vi "Read Channel Names.vi"(8 "error in (no error)":errorcluster, 11 "Temp Control in":refnum<class "Temp Control.lvclass">) -> (0 "error out":errorcluster, 2 "Channel Names":string[](array[string])=["Telescope RA", "Telescope DEC", "Telescope Moving?", "Telescope Status"], 3 "Temp Control out":refnum<class "Temp Control.lvclass">)   [LabVIEW 2022 SP3, in "Temp Control.lvclass"]
uses:
  Temp Control.lvclass
  Temp Control.lvclass/Temp Control.ctl
  hk-channel-class/hk-channel-class/HK Item/HK Item.lvclass
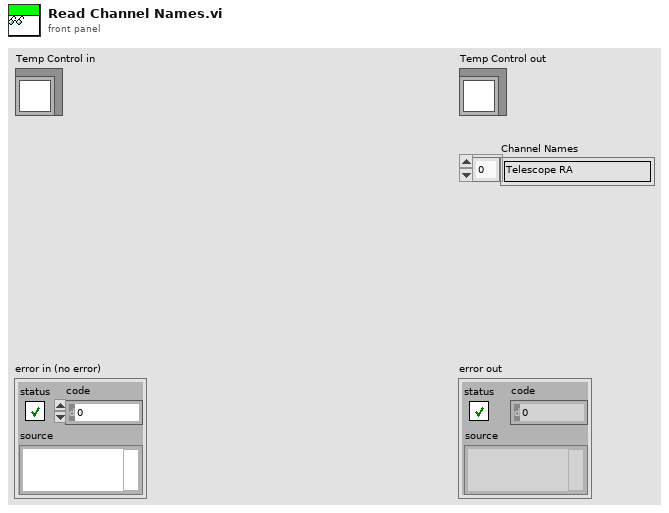
[diagram p1: front panel]
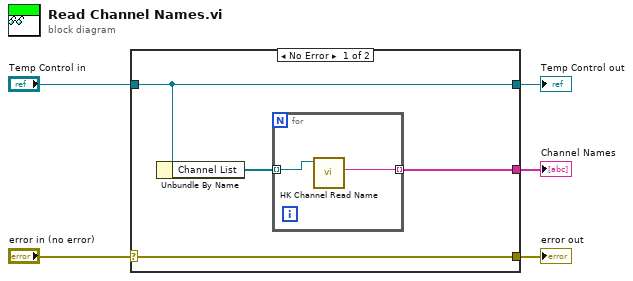
[diagram p0: block diagram]
diagram:
  n1 = case shown="No Error" "error in (no error)" {
    selector: "error in (no error)" -> [w9 w12]
    tunnel: [w9 w12] -> w4
    tunnel: [w8 w13] -> w2
    tunnel: "Temp Control in" -> [w8 w13]
    tunnel: [w6 _] -> w1
    frame No Error {
      n2 = Unbundle By Name(w8) -> ("Channel List"=w7:refnum<class "HK Item.lvclass">[])
      n3 = for {
        tunnel: w7 -> [w11] mode=indexing
        tunnel: [w10] -> w6 mode=indexing
        n4 = call "HK Channel Read Name.vi"("HK Item in"=w11) -> ("Name"=w10:string)  [unwired: 8 in, 2 out]
      }
    }
    frame Error {
    }
  }
  "error out" <- w4
  "Temp Control out" <- w2
  "Channel Names" <- w1
